vi "POLARIS Focus Camera.vi"() -> ()   [LabVIEW 2009]
uses:
  <vilib>/userDefined/High Color/IMAQdx.ctl
  XDisplay/POLARIS IMAQ Display.xctl
  Analyze Classes/Width Method.ctl
  IMAQdx Cam/IMAQdx Cam.lvclass
  XDisplay/Properties/ImageSource.ctl
  Analyze Classes/Analyze Q-Factor/Analyze q-Factor.lvclass
  Analyze Classes/Analyze Fluence/Analyze Fluence.lvclass
  Utility/POLARIS Vision utility.lvlib
panel:
  in  "SW Trigger":bool
  out "error out":errorcluster
  out "q-Factor":dbl format="%#_3g"
  out "Focus/µm^2":dbl
  in  "Method":T1
  in  "Size of hotest Region":i32=10
  in  "Energy [J]":dbl=10.0
  out "error save settings":errorcluster
  in  "Config Dir":path=path "D:/Test XDisplay images"
  in  "Prefix":string
  in  "WorkDir":path=path "D:/Test XDisplay images"
  out "XDisplay":cluster{"Image":T2}(xcontrol)
  in  "stop":bool
  in  "Camera Name":T3="JustageCam"
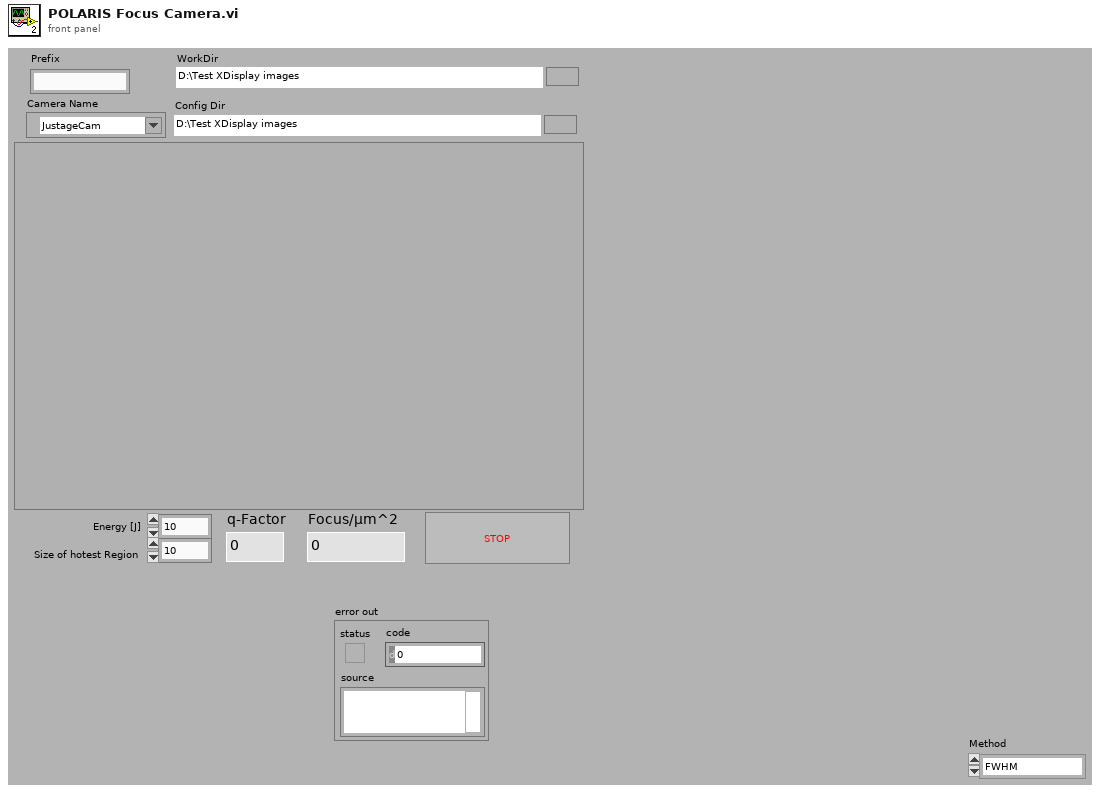
[diagram p1: front panel]
types:
  T1 = typedef "Width Method.ctl" = enum16{"FWHM", "1/e", "1/e^2", "80%", "90%"}
  T2 = typedef "IMAQ Image.ctl" = refnum<image>
  T3 = typedef "IMAQdx.ctl" = refnum<k21>
  T4 = typedef "Image Type" = u32
  T5 = typedef "POLARIS IMAQ Display.xctl/ImageSource.ctl" = enum16{"Camera", "File"}
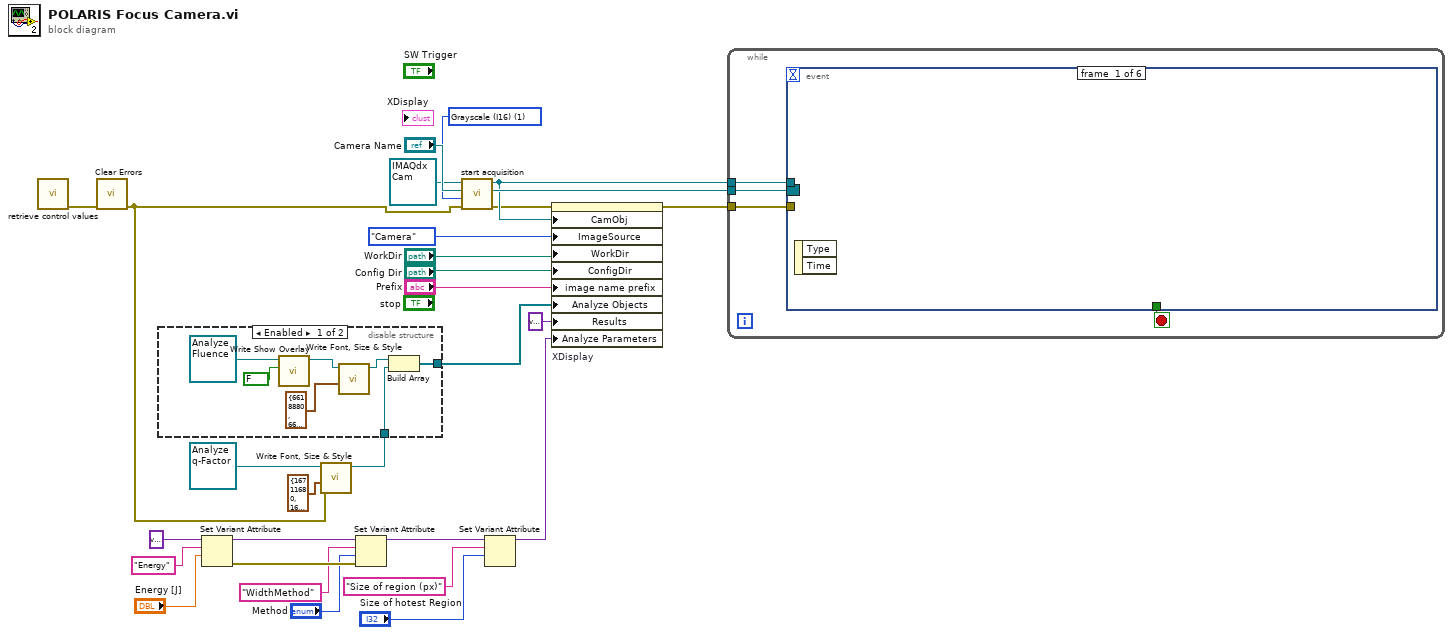
[diagram p0: block diagram]
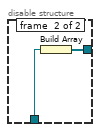
[diagram p2: hidden frame]
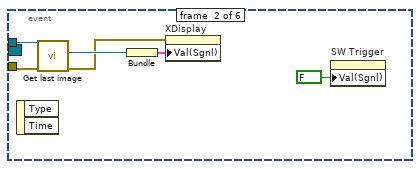
[diagram p3: hidden frame]
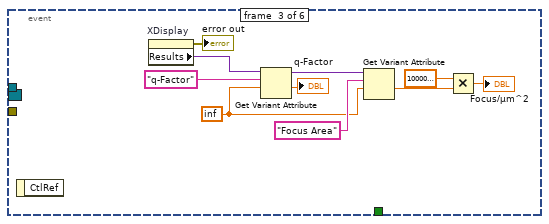
[diagram p4: hidden frame]
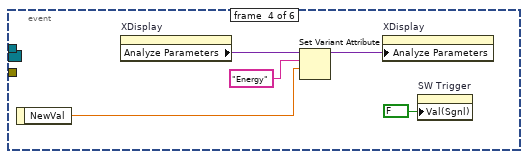
[diagram p5: hidden frame]
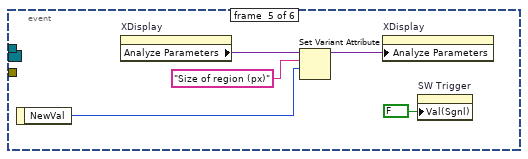
[diagram p6: hidden frame]
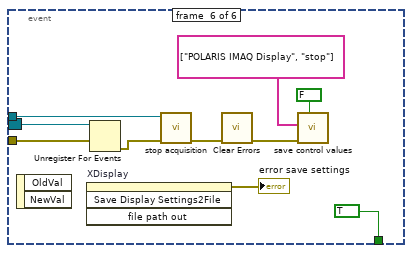
[diagram p7: hidden frame]
diagram:
  w21 = T4 1 items=["Grayscale (U8)", "Grayscale (I16)", "Grayscale (SGL)", "Complex (CSG)", "RGB (U32)", "HSL (U32)", "RGB (U64)", "Grayscale (U16)"] ("Image Type")
  n1 = call "retrieve control values.vi"() -> ("error out"=w18:errorcluster)  [unwired: 10 in, 1 out]
  n2 = call <vilib>:"Clear Errors.vi"("error in (no error)"=w18) -> ("error out"=w12:errorcluster)  [unwired: 6 in]
  n3 = Set Variant Attribute(Variant=variant ("variant"), name="Energy", value="Energy [J]") -> (Variant out=w9:variant, error out=w11:errorcluster)  [unwired: 1 in, 1 out]
  n4 = call-dynamic "Write Font, Size & Style.vi"("error in (no error)"=w12, "Overlay colors"=cluster{"Border":u32, "Text":u32} {"Border"=16711680, "Text"=16448250}, "Analyze BaseClass in"=refnum<class "Analyze q-Factor.lvclass"> refnum ("Analyze Q-Factor.lvclass")) -> ("Analyze BaseClass out"=w15:refnum<class "Analyze q-Factor.lvclass">)  [unwired: 7 in, 1 out]
  n5 = disable-structure shown="Enabled" {
    disable-tunnel: [w36 w37] -> w14
    disable-tunnel: w15 -> [w35 w38]
    frame #0 {
      n6 = call-dynamic "Write Show Overlay.vi"("Overlay?"=FALSE, "Analyze BaseClass in"=refnum<class "Analyze Fluence.lvclass"> refnum ("Analyze Fluence.lvclass")) -> ("Analyze BaseClass out"=w31:refnum<class "Analyze Fluence.lvclass">)  [unwired: 8 in, 1 out]
      n7 = call-dynamic "Write Font, Size & Style.vi"("Overlay colors"=cluster{"Border":u32, "Text":u32} {"Border"=6618880, "Text"=6618880}, "Analyze BaseClass in"=w31) -> ("Analyze BaseClass out"=w30:refnum<class "Analyze Fluence.lvclass">)  [unwired: 8 in, 1 out]
      n8 = Build Array(w30, w35) -> (w36:refnum<class "Analyze BaseClass.lvclass">[])
    }
    frame #1 {
      n9 = Build Array(w38) -> (w37:refnum<class "Analyze q-Factor.lvclass">[])
    }
  }
  n10 = Set Variant Attribute(Variant=w9, name="WidthMethod", value="Method", error in=w11) -> (Variant out=w4:variant)  [unwired: 2 out]
  n11 = call-dynamic "start acquisition.vi"("error in (no error)"=w12, "Image Type"=w21, "Camera Name"="Camera Name", "IMAQdx Cam in"=refnum<class "IMAQdx Cam.lvclass"> refnum ("IMAQdx Cam.lvclass")) -> ("error out"=w23:errorcluster, "Event Registration Refnum"=w28:refnum<event-registration>, "IMAQdx Cam out"=w24:refnum<class "IMAQdx Cam.lvclass">)  [unwired: 5 in]
  n12 = Set Variant Attribute(Variant=w4, name="Size of region (px)", value="Size of hotest Region") -> (Variant out=w3:variant)  [unwired: 1 in, 2 out]
  n13 = property on="XDisplay" class="POLARIS IMAQ Display (strict)"(error in=w23, "CamObj"=w24, "ImageSource"=ImageSource."Camera", "WorkDir"="WorkDir", "ConfigDir"="Config Dir", "image name prefix"="Prefix", "Analyze Objects"=w14, "Results"=variant, "Analyze Parameters"=w3) -> (error out=w22:errorcluster)  [unwired: 1 in, 1 out]
  n14 = while {
    tunnel: w24 -> [w41]
    tunnel: w28 -> [w40]
    tunnel: w22 -> [w39]
    stop <- w42 stop-if-true
    n15 = event shown="[4] \"Size of hotest Region\": Value Change" {
      selector: w40 -> [_ _ _ _ _ w75]
      dyn-events: _ -> [_ _ _ _ _ _]
      timeout: _ -> [_ _ _ _ _ _]
      tunnel: [_ _ _ _ _ TRUE] -> w42
      tunnel: w41 -> [_ w48 _ _ _ w76]
      tunnel: w39 -> [_ w47 _ _ _ w74]
      event #0 {
        n16 = event-data() -> ()  [unwired: 1 in, 2 out]
      }
      event #1 {
        n17 = event-data() -> ()  [unwired: 1 in, 2 out]
        n18 = call-dynamic "Get last image.vi"("error in (no error)"=w47, "IMAQdx Cam in"=w48) -> ("error out"=w45:errorcluster, "Image Out"=w46:T2)  [unwired: 7 in, 1 out]
        n19 = Bundle("Image Out"=w46) -> (w44:cluster{"Image Out":T2})  [unwired: 1 in]
        n20 = property on="XDisplay" class="POLARIS IMAQ Display (strict)"(error in=w45, "Val(Sgnl)"=w44) -> ()  [unwired: 1 in, 2 out]
        n21 = property on="SW Trigger" class="Bool (strict)"("Val(Sgnl)"=FALSE ("Value (Signaling)")) -> ()  [unwired: 2 in, 2 out]
      }
      event #2 {
        w53 = inf
        n22 = event-data() -> ()  [unwired: 1 in, 1 out]
        n23 = property on="XDisplay" class="POLARIS IMAQ Display (strict)"() -> (error out=→"error out":errorcluster, "Results"=w57:variant)  [unwired: 2 in, 1 out]
        n24 = Get Variant Attribute(Variant=w57, name="q-Factor", default value (empty Variant)=w53) -> (duplicate Variant=w54:variant, value=→"q-Factor":dbl)  [unwired: 1 in, 2 out]
        n25 = Get Variant Attribute(Variant=w54, name="Focus Area", default value (empty Variant)=w53) -> (value=w52:dbl)  [unwired: 1 in, 3 out]
        n26 = Multiply(x=1000000.0, y=w52) -> (x*y=→"Focus/µm^2":dbl)
      }
      event #3 {
        n27 = event-data() -> ("NewVal"=w60:dbl)  [unwired: 1 in]
        n28 = property on="XDisplay" class="POLARIS IMAQ Display (strict)"() -> ("Analyze Parameters"=w63:variant)  [unwired: 2 in, 2 out]
        n29 = Set Variant Attribute(Variant=w63, name="Energy", value=w60) -> (Variant out=w61:variant)  [unwired: 1 in, 2 out]
        n30 = property on="XDisplay" class="POLARIS IMAQ Display (strict)"("Analyze Parameters"=w61) -> ()  [unwired: 2 in, 2 out]
        n31 = property on="SW Trigger" class="Bool (strict)"("Val(Sgnl)"=FALSE ("Value (Signaling)")) -> ()  [unwired: 2 in, 2 out]
      }
      event #4 {
        n32 = event-data() -> ("NewVal"=w65:i32)  [unwired: 1 in]
        n33 = property on="XDisplay" class="POLARIS IMAQ Display (strict)"() -> ("Analyze Parameters"=w68:variant)  [unwired: 2 in, 2 out]
        n34 = Set Variant Attribute(Variant=w68, name="Size of region (px)", value=w65) -> (Variant out=w66:variant)  [unwired: 1 in, 2 out]
        n35 = property on="XDisplay" class="POLARIS IMAQ Display (strict)"("Analyze Parameters"=w66) -> ()  [unwired: 2 in, 2 out]
        n36 = property on="SW Trigger" class="Bool (strict)"("Val(Sgnl)"=FALSE ("Value (Signaling)")) -> ()  [unwired: 2 in, 2 out]
      }
      event #5 {
        n37 = event-data() -> ()  [unwired: 1 in, 2 out]
        n38 = invoke on="XDisplay" class="POLARIS IMAQ Display (strict)" method="Save Display Settings2File"() -> (error out=→"error save settings":errorcluster)  [unwired: 4 in, 3 out]
        n39 = Unregister For Events(event registration refnum=w75, error in=w74) -> (error out=w77:errorcluster)
        n40 = call-dynamic "stop acquisition.vi"("error in (no error)"=w77, "IMAQdx Cam in"=w76) -> ("error out"=w73:errorcluster)  [unwired: 8 in, 1 out]
        n41 = call <vilib>:"Clear Errors.vi"("error in (no error)"=w73) -> ("error out"=w72:errorcluster)  [unwired: 6 in]
        n42 = call "save control values.vi"("Append timestamp (true)"=FALSE, "error in"=w72, "Dont save"=string[] ["POLARIS IMAQ Display", "stop"]) -> ()  [unwired: 5 in, 2 out]
      }
    }
  }
